vi "FS-Packet over Ethernet Duplex.vi"() -> ()   [LabVIEW 2020]
uses:
  FGV Mode.ctl
  <vilib>/Utility/error.llb/DialogType.ctl
  <instrlib>/niUSRP/niUSRP Write Tx Data (I16).vi
  <instrlib>/niUSRP/niUSRP Fetch Rx Data (I16).vi
panel:
  in  "停止":bool
  out "UDP recv bytes":i32
  in  "UDP socket buffer size (recv)":i32=64000
  out "tx buffer (current)":i32
  out "rx buffer (current)":i32
  in  "tx gain":dbl format="%#_6f"
  out "UDP Recv timeout":bool
  out "usrp tx loop":errorcluster
  out "usrp rx loop":errorcluster
  in  "USRP送信用バッファサイズ":i32=500
  out "tx buffer full":bool caption="tx buffer full (UDP - USRP)"
  in  "srcport":i32=40000 caption="IQデータを受信するポート番号"
  in  "srcaddr":string="192.168.0.109" caption="IQデータを受信するIPアドレス"
  out "rx buffer full":bool caption="rx buffer full (USRP - UDP)"
  in  "rx buff size (max)":i32=500 caption="USRP受信用バッファサイズ"
  in  "dsrport":i32=40000 caption="IQデータ送信先のポート番号"
  in  "dstaddr":string="192.168.0.112" caption="IQデータ送信先のIPアドレス"
  out "data":i16[](array[numeric])
  in  "rx gain":dbl format="%#_6f"
  in  "carrier frequency":dbl=2000000000.0 format="%#_6p"
  in  "IQ rate":dbl=100000.0 format="%#_6p"
  in  "number of samples":i64=2000
  in  "device names":refnum<k15>="192.168.1.51"
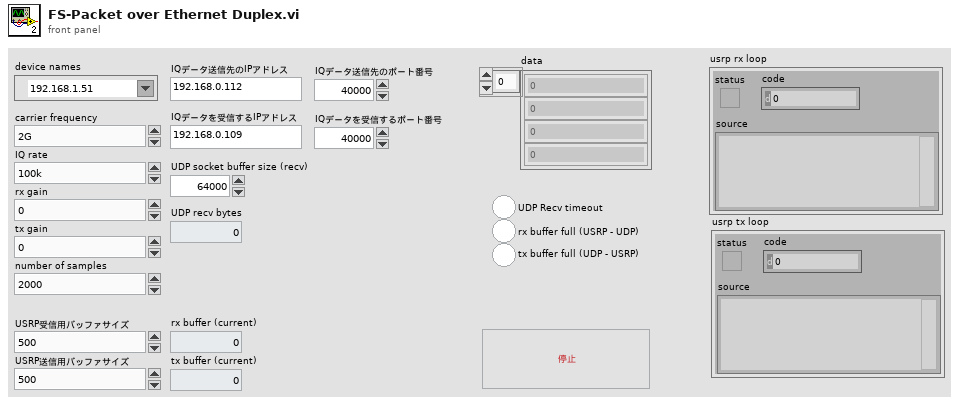
[diagram p1: front panel]
types:
  T1 = typedef "FGV Mode.ctl" = enum16{"None", "Init", "Set", "Get", "Update", "Clear"}
  T2 = typedef "DialogType.ctl" = u16
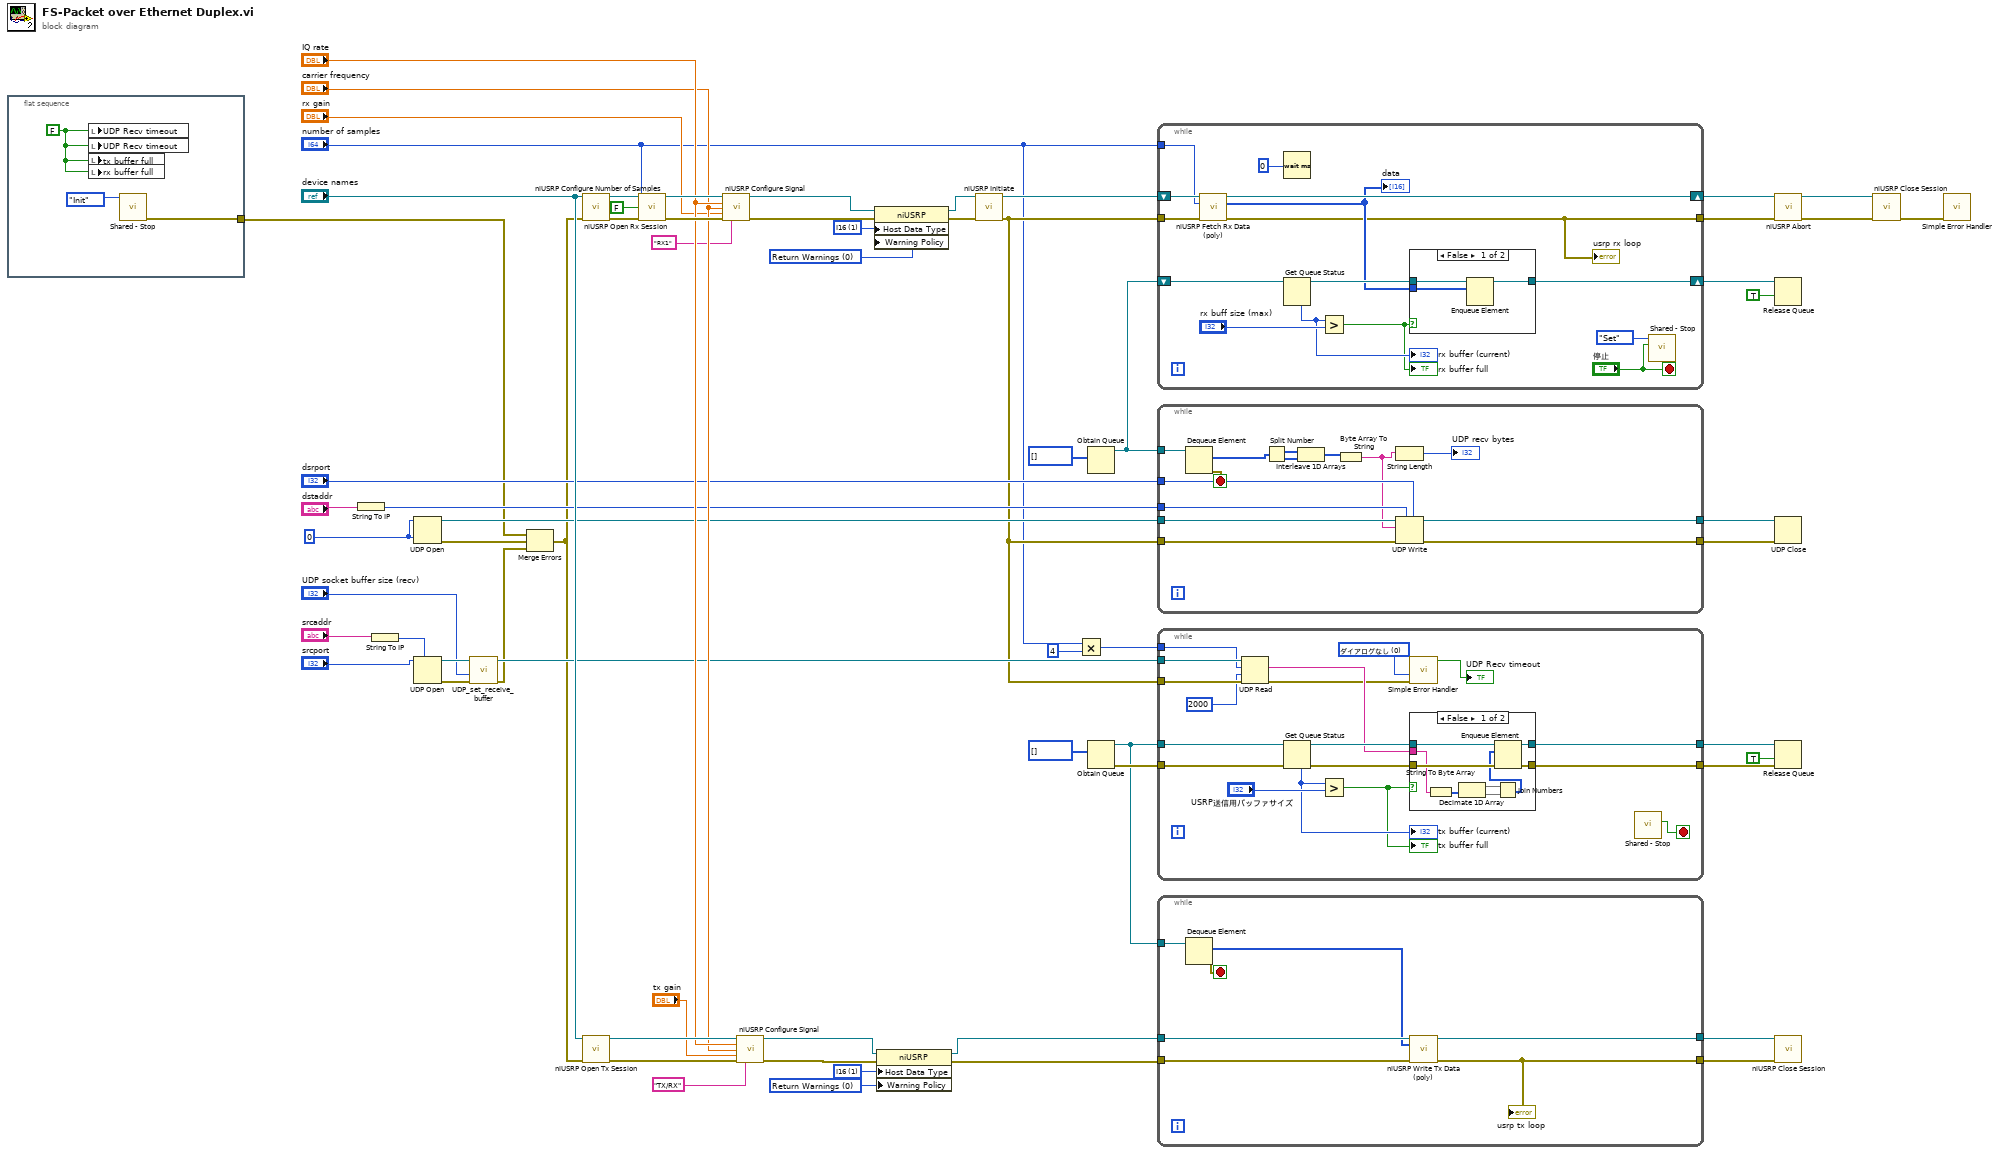
[diagram p0: block diagram]
diagram:
  w27 = u32 0 ("ネットアドレス")
  w36 = 0 items=["Return Warnings", "Return Errors", "Return Success"] ("Configuration:Advanced:Warning Policy")
  w37 = 1 items=["CDB", "I16"] ("Configuration:Advanced:Host Data Type")
  w42 = 0 items=["Return Warnings", "Return Errors", "Return Success"] ("Configuration:Advanced:Warning Policy")
  w43 = 1 items=["CDB", "I16"] ("Configuration:Advanced:Host Data Type")
  n1 = flat-sequence {
    tunnel: [w67] -> w3
    frame #0 {
      w69 = FALSE ("USRP rx overflow")
      n2 = local write "UDP Recv timeout"(w69) -> ()
      n3 = local write "UDP Recv timeout"(w69) -> ()
      n4 = local write "tx buffer full"(w69) -> ()
      n5 = local write "rx buffer full"(w69) -> ()
      n6 = call "Shared - Stop.vi"("FGV Mode"=FGV_Mode."Init") -> ("error out"=w67:errorcluster)  [unwired: 9 in, 1 out]
    }
  }
  n7 = String To IP(1:"dstaddr") -> (0:w29:u32)
  n8 = String To IP(1:"srcaddr") -> (0:w23:u32)
  n9 = UDP Open(7:w27, 11:w27) -> (port=w32:refnum<k16>, 0:w11:errorcluster)  [unwired: 3 in, 1 out]
  n10 = UDP Open(7:w23, 11:"srcport") -> (port=w16:refnum<k16>, 0:w15:errorcluster)  [unwired: 3 in, 1 out]
  n11 = call "UDP_set_receive_buffer.vi"("error in (no error)"=w15, "Receive Buffer Size"="UDP socket buffer size (recv)", "connection ID"=w16) -> ("error out"=w2:errorcluster, "connection ID out"=w14:refnum<k16>)  [unwired: 6 in]
  n12 = Merge Errors(w3, w11, w2) -> (w1:errorcluster)
  n13 = call <instrlib>:"niUSRP Open Rx Session.vi"("device names"="device names", "error in (no error)"=w1) -> ("session handle out"=w66:refnum<k15>, "error out"=w57:errorcluster)  [unwired: 12 in]
  n14 = call <instrlib>:"niUSRP Open Tx Session.vi"("device names"="device names", "error in (no error)"=w1) -> ("session handle out"=w54:refnum<k15>, "error out"=w53:errorcluster)  [unwired: 12 in]
  n15 = call <instrlib>:"niUSRP Configure Number of Samples.vi"("session handle"=w66, "number of samples is finite"=FALSE, "number of samples"="number of samples", "error in (no error)"=w57) -> ("session handle out"=w65:refnum<k15>, "error out"=w58:errorcluster)  [unwired: 10 in]
  n16 = call <instrlib>:"niUSRP Configure Signal.vi"("session handle"=w65, "IQ rate"="IQ rate", "carrier frequency"="carrier frequency", "gain"="rx gain", "error in (no error)"=w58, "active antenna"="RX1") -> ("session handle out"=w64:refnum<k15>, "error out"=w44:errorcluster)  [unwired: 5 in, 3 out]
  n17 = call <instrlib>:"niUSRP Configure Signal.vi"("session handle"=w54, "IQ rate"="IQ rate", "carrier frequency"="carrier frequency", "gain"="tx gain", "error in (no error)"=w53, "active antenna"="TX/RX") -> ("session handle out"=w41:refnum<k15>, "error out"=w39:errorcluster)  [unwired: 5 in, 3 out]
  n18 = property class="niUSRP"(reference=w64, error in=w44, "Host Data Type"=w43, "Warning Policy"=w42) -> (reference out=w45:refnum<k15>, error out=w10:errorcluster)
  n19 = property class="niUSRP"(reference=w41, error in=w39, "Host Data Type"=w37, "Warning Policy"=w36) -> (reference out=w40:refnum<k15>, error out=w38:errorcluster)
  n20 = call <instrlib>:"niUSRP Initiate.vi"("session handle"=w45, "error in (no error)"=w10) -> ("session handle out"=w63:refnum<k15>, "error out"=w9:errorcluster)  [unwired: 12 in]
  n21 = Multiply(x="number of samples", y=4 ("最大サイズ (548)")) -> (x*y=w6:i64)
  n22 = Obtain Queue(element data type=i16[] []) -> (queue out=w33:refnum<queue>)  [unwired: 4 in, 2 out]
  n23 = Obtain Queue(element data type=i16[] []) -> (queue out=w17:refnum<queue>, error out=w21:errorcluster)  [unwired: 4 in, 1 out]
  n24 = while {
    shift-right: [w83] -> w62
    shift-left: w63 -> [w84]
    tunnel: "number of samples" -> [w80]
    shift-right: [w79] -> w31
    shift-left: w33 -> [w78]
    tunnel: w9 -> [w82]
    tunnel: [w70] -> w59
    stop <- "停止" stop-if-true
    n25 = call-poly <instrlib>:"niUSRP Fetch Rx Data (poly).vi"("session handle"=w84, "number of samples"=w80, "error in (no error)"=w82) -> ("session handle out"=w83:refnum<k15>, "data"=w75:i16[], "error out"=w70:errorcluster)  [unwired: 9 in, 1 out]
    "data" <- w75
    "usrp rx loop" <- w70
    n26 = Wait (ms)(milliseconds to wait=u32 0 ("ミリ秒待機時間")) -> ()  [unwired: 1 out]
    n27 = Get Queue Status(queue=w78) -> (queue out=w77:refnum<queue>, # elements in queue=w73:i32)  [unwired: 2 in, 6 out]
    "rx buffer (current)" <- w73
    n28 = Greater?(x=w73, y="rx buff size (max)") -> (0:w72:bool)
    "rx buffer full" <- w72
    n29 = case shown="FALSE" w72 {
      tunnel: [w87 w88] -> w79
      tunnel: w77 -> [w86 w88]
      tunnel: w75 -> [w85 _]
      frame False {
        n30 = Enqueue Element(queue=w86, element=w85) -> (queue out=w87:refnum<queue>)  [unwired: 2 in, 2 out]
      }
      frame True {
      }
    }
    n31 = call "Shared - Stop.vi"("Stop in"="停止", "FGV Mode"=FGV_Mode."Set") -> ()  [unwired: 8 in, 2 out]
  }
  n32 = while {
    tunnel: w33 -> [w102]
    tunnel: w32 -> [w100]
    tunnel: w29 -> [w95]
    tunnel: "dsrport" -> [w94]
    tunnel: w9 -> [w93]
    tunnel: [w92] -> w26
    tunnel: [w91] -> w25
    stop <- w101 stop-if-true
    n33 = Dequeue Element(queue=w102) -> (element=w99:i16[], error out=w101:errorcluster)  [unwired: 2 in, 2 out]
    n34 = Split Number(x=w99) -> (hi(x)=w98:u8[], lo(x)=w97:u8[])
    n35 = Interleave 1D Arrays(w98, w97) -> (w96:u8[])
    n36 = Byte Array To String(unsigned byte array=w96) -> (string=w90:string)
    n37 = String Length(string=w90) -> (length=→"UDP recv bytes":i32)
    n38 = UDP Write(address=w95, port or service name=w94, connection ID=w100, data in=w90, 8:w93) -> (error out=w91:errorcluster, 3:w92:refnum<k16>)  [unwired: 1 in]
  }
  n39 = while {
    tunnel: w14 -> [w120]
    tunnel: w9 -> [w119]
    tunnel: w17 -> [w117]
    tunnel: w21 -> [w116]
    tunnel: [w113] -> w19
    tunnel: [w111] -> w18
    tunnel: w6 -> [w108]
    stop <- w110 stop-if-true
    w105 = T2 0 items=["ダイアログなし", "OKメッセージ", "継続か停止メッセージ", "OKメッセージ+警告", "継続/停止+警告"] ("type of dialog (OK msg:1)")
    n40 = UDP Read(connection ID=w120, max size (548)=w108, timeout ms (25000)=2000 ("タイムアウト (ms) (25000)"), 8:w119) -> (data out=w115:string, error out=w107:errorcluster)  [unwired: 3 out]
    n41 = Get Queue Status(queue=w117, error in (no error)=w116) -> (queue out=w118:refnum<queue>, error out=w112:errorcluster, # elements in queue=w104:i32)  [unwired: 1 in, 5 out]
    "tx buffer (current)" <- w104
    n42 = Greater?(x=w104, y="USRP送信用バッファサイズ") -> (0:w103:bool)
    "tx buffer full" <- w103
    n43 = call <vilib>:"Simple Error Handler.vi"("type of dialog (OK msg:1)"=w105, "error in (no error)"=w107) -> ("error?"=→"UDP Recv timeout":bool)  [unwired: 3 in, 4 out]
    n44 = case shown="FALSE" w103 {
      tunnel: [w129 w131] -> w113
      tunnel: w118 -> [w128 w131]
      tunnel: w115 -> [w122 _]
      tunnel: w112 -> [w127 w130]
      tunnel: [w126 w130] -> w111
      frame False {
        n45 = String To Byte Array(string=w122) -> (unsigned byte array=w123:u8[])
        n46 = Decimate 1D Array(w123) -> (w124:u8[], w125:u8[])
        n47 = Join Numbers(hi=w124, lo=w125) -> ((hi.lo)=w121:u16[])
        n48 = Enqueue Element(queue=w128, element=w121, error in (no error)=w127) -> (queue out=w129:refnum<queue>, error out=w126:errorcluster)  [unwired: 1 in, 1 out]
      }
      frame True {
      }
    }
    n49 = call "Shared - Stop.vi"() -> ("Stop out"=w110:bool)  [unwired: 10 in, 1 out]
  }
  n50 = while {
    tunnel: w40 -> [w138]
    tunnel: w38 -> [w137]
    tunnel: [w136] -> w48
    tunnel: [w132] -> w47
    tunnel: w17 -> [w135]
    stop <- w134 stop-if-true
    n51 = Dequeue Element(queue=w135) -> (element=w133:i16[], error out=w134:errorcluster)  [unwired: 2 in, 2 out]
    n52 = call-poly <instrlib>:"niUSRP Write Tx Data (poly).vi"("session handle"=w138, "data"=w133, "error in (no error)"=w137) -> ("session handle out"=w136:refnum<k15>, "error out"=w132:errorcluster)  [unwired: 11 in]
    "usrp tx loop" <- w132
  }
  n53 = call <instrlib>:"niUSRP Abort.vi"("session handle"=w62, "error in (no error)"=w59) -> ("session handle out"=w61:refnum<k15>, "error out"=w60:errorcluster)  [unwired: 12 in]
  n54 = Release Queue(queue=w31, force destroy? (F)=TRUE ("破棄を強制? (F)")) -> ()  [unwired: 1 in, 3 out]
  n55 = UDP Close(connection ID=w26, 8:w25) -> ()  [unwired: 2 out]
  n56 = Release Queue(queue=w19, force destroy? (F)=TRUE ("破棄を強制? (F)"), error in (no error)=w18) -> ()  [unwired: 3 out]
  n57 = call <instrlib>:"niUSRP Close Session.vi"("session handle"=w48, "error in (no error)"=w47) -> ()  [unwired: 13 in, 1 out]
  n58 = call <instrlib>:"niUSRP Close Session.vi"("session handle"=w61, "error in (no error)"=w60) -> ("error out"=w13:errorcluster)  [unwired: 13 in]
  n59 = call <vilib>:"Simple Error Handler.vi"("error in (no error)"=w13) -> ()  [unwired: 4 in, 5 out]
